vi "ToTable.vi"(8 "error in (no error)":errorcluster, 9 "Table Index":i32, 10 "variant":variant, 11 "Scaling editor node in":refnum<class "Scaling editor node.lvclass">) -> (0 "error out":errorcluster, 1 "row header":string[](array[string]), 2 "table":string[][](array[string]), 3 "Scaling editor node out":refnum<class "Scaling editor node.lvclass">)   [LabVIEW 2013, in "Scaling editor node.lvclass"]
uses:
  Scaling editor node.lvclass
  module/configuration/Scaling configuration.lvclass
  <vilib>/NI/Module Execution Interface/Engine Configuration/engine configuration.lvclass
  Scaling editor node.lvclass/Scaling editor node.ctl
  <vilib>/NI/Configuration Framework/serializable configuration/NISE_CEF_serializable configuration.lvclass/NISE_CEF_serializable configuration.ctl
  <vilib>/NI/Tag Bus/tag/tag descriptor.lvclass/tag descriptor.ctl
  <vilib>/Utility/LVClass/Get LV Class Name.vi
  <vilib>/NI/Configuration Framework/error generator/NISE_error generator.vi
  <vilib>/NI/Tag Bus/tag/tag descriptor.lvclass
  <vilib>/NI/Configuration Framework/serializable configuration/NISE_CEF_serializable configuration.lvclass
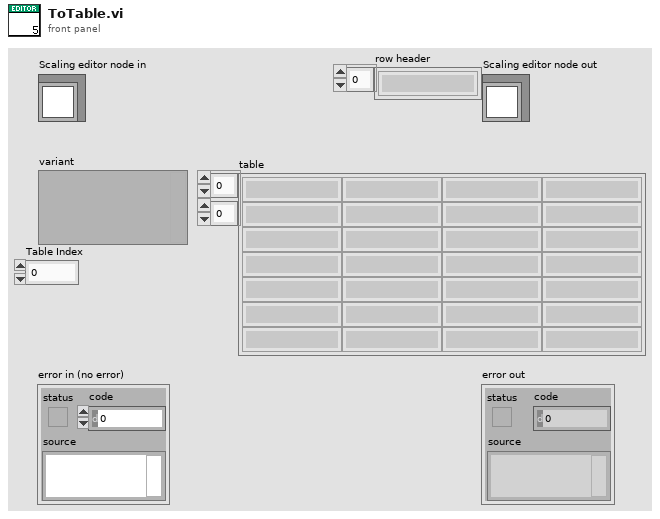
[diagram p1: front panel]
types:
  T1 = typedef "Scaling configuration.lvclass/scale data types.ctl" = enum16{"Double", "Single", "I64", "I32", "I16", "I8", "U64", "U32", "U16", "U8", "Boolean"}
  T2 = cluster{"input channel":refnum<class "TBM channel.lvclass">, "output channel":refnum<class "TBM channel.lvclass">, "input data type":T1, "output data type":T1}[]
  T3 = typedef "tag bus.lvlib/tag descriptor.lvclass/Data Type.ctl" = enum16{"Double", "Single", "I64", "I32", "I16", "I8", "U64", "U32", "U16", "U8", "Boolean", "String", "Array of Double", "Array of Single", "Array of I64", "Array of I32", "Array of I16", "Array of I8", "Array of U64", "Array of U32", "Array of U16", "Array of U8", "Array of Boolean", "Array of String"}
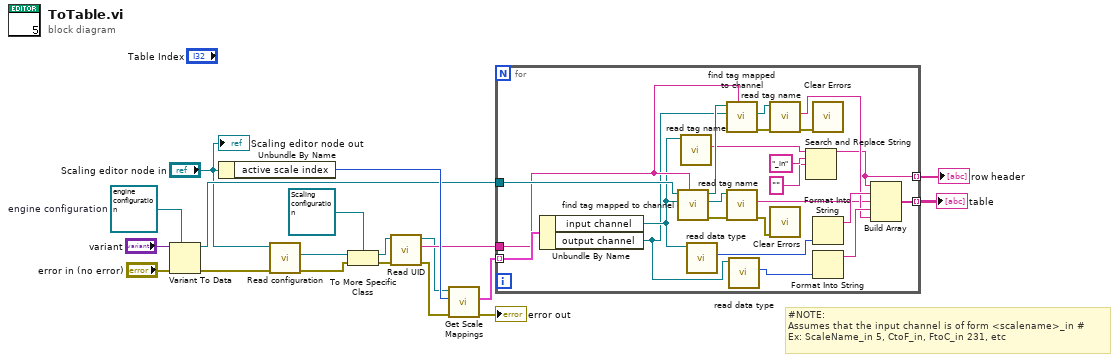
[diagram p0: block diagram]
diagram:
  w15 = refnum<class "engine configuration.lvclass"> refnum  # engine configuration
  # "#NOTE:\nAssumes that the input channel is of form <scalename>_in #\nEx: ScaleName_in 5, CtoF_in, FtoC_in 231, etc"
  n1 = Variant To Data(error in="error in (no error)", type=w15, Variant="variant") -> (data=w13:refnum<class "engine configuration.lvclass">, error out=w11:errorcluster)
  n2 = Unbundle By Name("Scaling editor node in") -> ("active scale index"=w16:i32)
  n3 = call-dynamic "Read configuration.vi"("error in"=w11, "Scaling editor node in"="Scaling editor node in") -> ("error out"=w17:errorcluster, "configuration"=w18:refnum<class "NISE_CEF_serializable configuration.lvclass">)  [unwired: 7 in, 1 out]
  n4 = To More Specific Class(target class=refnum<class "Scaling configuration.lvclass"> refnum ("Scaling configuration"), reference=w18, error in=w17) -> (specific class reference=w8:refnum<class "Scaling configuration.lvclass">, error out=w5:errorcluster)
  n5 = call <vilib>:"Read UID.vi"("error in"=w5, "configuration in"=w8) -> ("error out"=w4:errorcluster, "instance id"=w7:string, "configuration out"=w6:refnum<class "Scaling configuration.lvclass">)  [unwired: 7 in]
  n6 = call "Get Scale Mappings.vi"("error in (no error)"=w4, "index"=w16, "Scaling configuration in"=w6) -> ("error out"=→"error out":errorcluster, "mappings"=w10:T2)  [unwired: 6 in, 1 out]
  n7 = for {
    tunnel: w10 -> [w42] mode=indexing
    tunnel: w13 -> [w41]
    tunnel: [w34] -> w9 mode=indexing
    tunnel: w7 -> [w33]
    tunnel: [w20] -> w1 mode=indexing
    n8 = Unbundle By Name(w42) -> ("input channel"=w24:refnum<class "TBM channel.lvclass">, "output channel"=w22:refnum<class "TBM channel.lvclass">)
    n9 = call <vilib>:"find tag mapped to channel.vi"("owner"=w33, "channel"=w24, "engine configuration in"=w41) -> ("error out"=w39:errorcluster, "tag"=w40:refnum<class "tag descriptor.lvclass">, "engine configuration out"=w35:refnum<class "engine configuration.lvclass">)  [unwired: 6 in]
    n10 = call <vilib>:"read tag name.vi"("system tag in"=w24) -> ("name"=w25:string)  [unwired: 8 in, 2 out]
    n11 = call <vilib>:"read data type.vi"("system tag in"=w24) -> ("data type"=w23:T3)  [unwired: 8 in, 2 out]
    n12 = call <vilib>:"find tag mapped to channel.vi"("owner"=w33, "channel"=w22, "engine configuration in"=w35) -> ("error out"=w36:errorcluster, "tag"=w32:refnum<class "tag descriptor.lvclass">)  [unwired: 6 in, 1 out]
    n13 = call <vilib>:"read tag name.vi"("error in"=w39, "system tag in"=w40) -> ("error out"=w38:errorcluster, "name"=w28:string)  [unwired: 7 in, 1 out]
    n14 = call <vilib>:"read data type.vi"("system tag in"=w22) -> ("data type"=w21:T3)  [unwired: 8 in, 2 out]
    n15 = call <vilib>:"read tag name.vi"("error in"=w36, "system tag in"=w32) -> ("error out"=w37:errorcluster, "name"=w29:string)  [unwired: 7 in, 1 out]
    n16 = call <vilib>:"Clear Errors.vi"("error in (no error)"=w38) -> ()  [unwired: 6 in, 1 out]
    n17 = Search and Replace String(input string=w25, search string="_in", replace string="" ("replace string (\"\")")) -> (result string=w20:string)  [unwired: 5 in, 3 out]
    n18 = call <vilib>:"Clear Errors.vi"("error in (no error)"=w37) -> ()  [unwired: 6 in, 1 out]
    n19 = Format Into String(w23) -> (resulting string=w31:string)  [unwired: 3 in, 1 out]
    n20 = Format Into String(w21) -> (resulting string=w30:string)  [unwired: 3 in, 1 out]
    n21 = Build Array(w20, w31, w28, w30, w29) -> (w34:string[])
  }
  "table" <- w9
  "row header" <- w1
  "Scaling editor node out" <- "Scaling editor node in"
